vi "Path as Encoded Path (UTF-8 Path).vi"(9 "error in":errorcluster, 10 "Path":refnum<class "UTF-8 Path.lvclass">) -> (1 "error out":errorcluster, 2 "Encoded Path":T1)   [LabVIEW 2020, in "G-Unicode.lvlib"]
doc: "Converts the input path to a raw UTF-8 encoded LabVIEW path. Valid inputs are a UTF-8 Path class or LabVIEW path."
uses:
  G-Unicode.lvlib
  Types/Encoded UTF-8 Path.ctl
  Types/UTF-8 Path/UTF-8 Path.lvclass
  Types/UTF-8 Path/UTF-8 Path.lvclass/UTF-8 Path.ctl
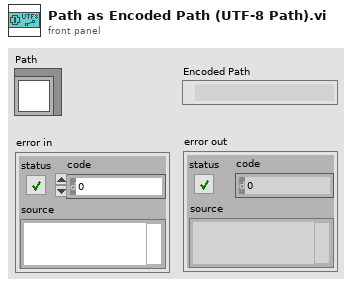
[diagram p1: front panel]
types:
  T1 = typedef "G-Unicode.lvlib/Encoded UTF-8 Path.ctl" = path
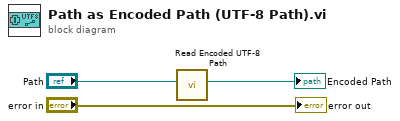
[diagram p0: block diagram]
diagram:
  n1 = call "Read Encoded UTF-8 Path.vi"("UTF-8 Path"="Path") -> ("Encoded UTF-8 Path"=→"Encoded Path":T1)  [unwired: 10 in]
  "error out" <- "error in"
